vi "Start Acquisition Temp File.vi"(8 "error in (no error)":errorcluster, 10 "Type":string) -> (0 "error out":errorcluster, 3 "Byte Stream File Refnum":refnum<file>)   [LabVIEW 2009]
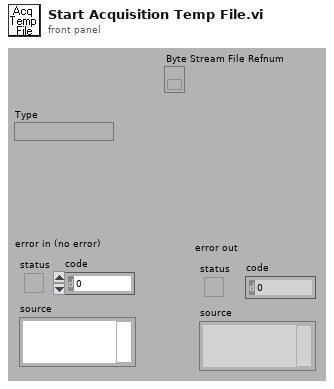
[diagram p1: front panel]
types:
  T1 = enum16{"open", "replace", "create", "open or create", "replace or create", "replace or create with confirmation"}
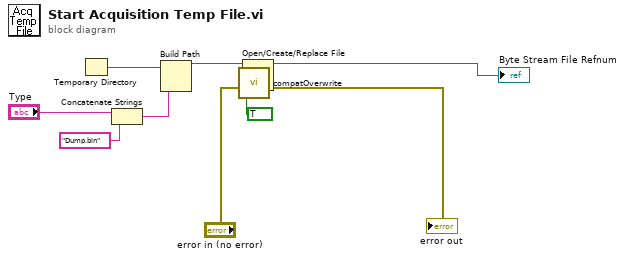
[diagram p0: block diagram]
diagram:
  n1 = Temporary Directory() -> (w7:path)
  n2 = Concatenate Strings("Type", "Dump.bin" ("Substring")) -> (w5:string)
  n3 = Build Path(base path=w7, name or relative path=w5) -> (appended path=w8:path)
  n4 = call <vilib>:"compatOverwrite.vi"("overwrite (F)"=TRUE) -> ("overwrite?"=w1:T1)
  n5 = Open/Create/Replace File(file path (use dialog)=w8, error in="error in (no error)", operation (0:open)=w1) -> (refnum out=→"Byte Stream File Refnum":refnum<file>, error out=→"error out":errorcluster)  [unwired: 3 in, 1 out]
